vi "Assert Array Equivalent.vi"(4 "Execution time (s)":dbl=-1.0, 5 "Assert Only? (F)":bool, 6 "error code (1)":i32=1, 7 "Label (\"\")":string, 8 "error in (no error)":errorcluster, 9 "Register with caller test (F)":bool, 10 "Second Array":variant, 11 "First Array":variant) -> (0 "error out":errorcluster, 2 "Properties.Assert":refnum<class "Properties.Assert.lvclass">)   [LabVIEW 2013, in "Caraya.lvlib" / "Assert.lvclass"]
doc: "Asserts that two arrays are equivalent."
uses:
  Assert.lvclass
  Properties.Assert/Properties.Assert.lvclass
  Properties/Properties.lvclass
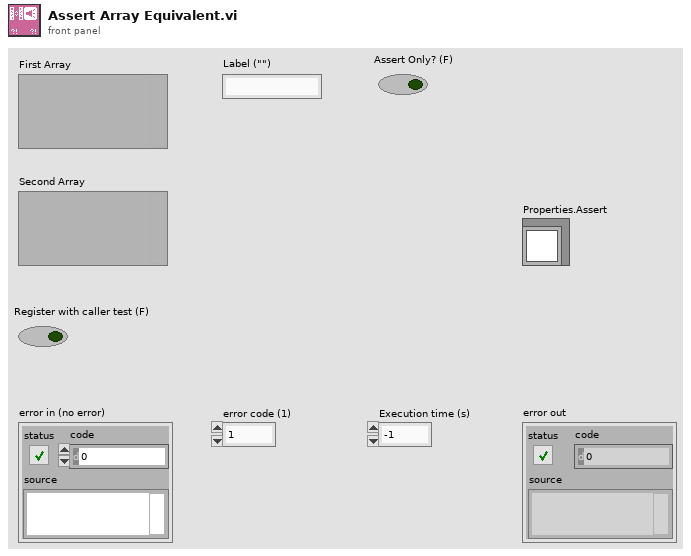
[diagram p1: front panel]
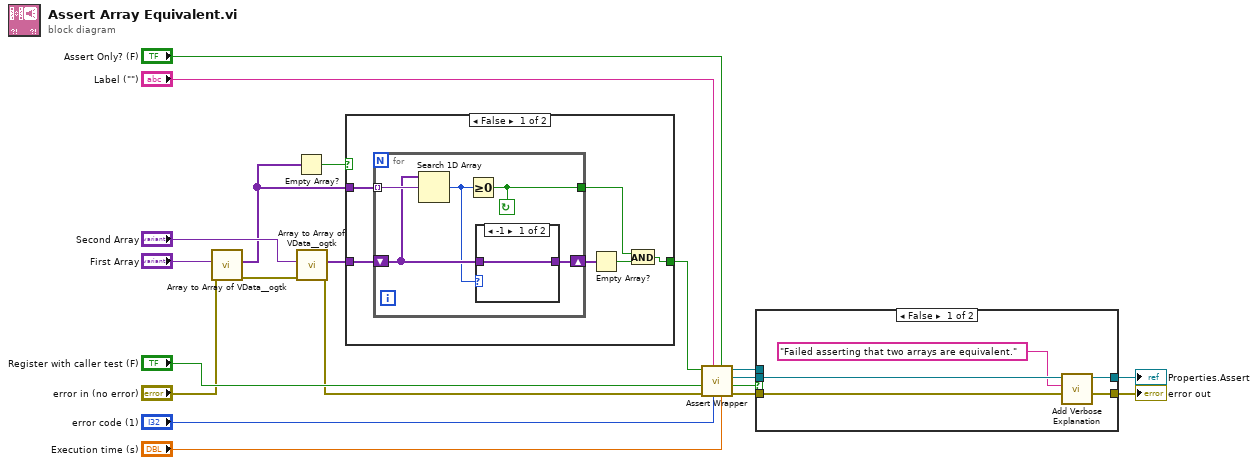
[diagram p0: block diagram]
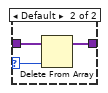
[diagram p2: hidden frame]
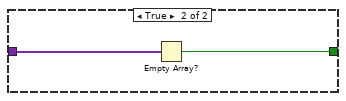
[diagram p3: hidden frame]
diagram:
  n1 = call <userlib>:"Array to Array of VData__ogtk.vi"("error in (no error)"="error in (no error)", "MultiD Array"="First Array") -> ("error out"=w7:errorcluster, "1D Array of Variants"=w2:variant[])  [unwired: 8 in]
  n2 = Empty Array?(array=w2) -> (empty?=w1:bool)
  n3 = call <userlib>:"Array to Array of VData__ogtk.vi"("error in (no error)"=w7, "MultiD Array"="Second Array") -> ("error out"=w6:errorcluster, "1D Array of Variants"=w4:variant[])  [unwired: 8 in]
  n4 = case shown="False" w1 {
    tunnel: w4 -> [w26 w37]
    tunnel: [w22 w36] -> w3
    tunnel: w2 -> [w21 _]
    frame False {
      n5 = for {
        shift-right: [w29] -> w25
        shift-left: w26 -> [w30]
        tunnel: w21 -> [w31] mode=indexing
        tunnel: [w28] -> w23
        stop <- w28 continue-if-true
        n6 = Search 1D Array(1D array=w30, element=w31) -> (index of element=w27:i32)  [unwired: 1 in]
        n7 = Greater Or Equal To 0?(x=w27) -> (x >= 0?=w28:bool)
        n8 = case shown="-1" w27 {
          selector: w27 -> [_ w33]
          tunnel: w30 -> [w32 w35]
          tunnel: [w32 w34] -> w29
          frame -1 {
          }
          frame Default {
            n9 = Delete From Array(array=w35, index=w33) -> (array with subset deleted=w34:variant[])  [unwired: 1 in, 1 out]
          }
        }
      }
      n10 = Empty Array?(array=w25) -> (empty?=w24:bool)
      n11 = And(x=w23, y=w24) -> (x .and. y?=w22:bool)
    }
    frame True {
      n12 = Empty Array?(array=w37) -> (empty?=w36:bool)
    }
  }
  n13 = call "Assert Wrapper.vi"("Execution time (s)"="Execution time (s)", "Assert Only? (F)"="Assert Only? (F)", "error code (1)"="error code (1)", "Label"="Label (\"\")", "error in (no error)"=w6, "Register with caller test (F)"="Register with caller test (F)", "Assert?"=w3) -> ("error out"=w11:errorcluster, "Verbose"=w15:bool, "Properties.Assert"=w13:refnum<class "Properties.Assert.lvclass">, "Assert out"=w14:refnum<class "Assert.lvclass">)  [unwired: 1 in]
  n14 = case shown="False" w15 {
    tunnel: w14 -> [_ _]
    tunnel: w13 -> [w40 w44]
    tunnel: [w41 w43] -> w12
    tunnel: w11 -> [w42 w43]
    tunnel: [w39 w44] -> w10
    frame False {
      n15 = call "Add Verbose Explanation.vi"("error in (no error)"=w42, "Verbose Explanation"="Failed asserting that two arrays are equivalent.", "Properties"=w40) -> ("error out"=w41:errorcluster, "Properties"=w39:refnum<class "Properties.Assert.lvclass">)  [unwired: 7 in]
    }
    frame True {
    }
  }
  "error out" <- w12
  "Properties.Assert" <- w10
